vi "CloseBling.vi"(5 "Turn off LEDs on close":bool=TRUE, 8 "error in (no error)":errorcluster, 11 "ControlState in":T1 {"ChainMask" format="0x%02x"}) -> (0 "error out":errorcluster)   [LabVIEW 2020, in "ArduinoSerialBling.lvlib"]
uses:
  ArduinoSerialBling.lvlib
  ControlState.ctl
  ChainState.ctl
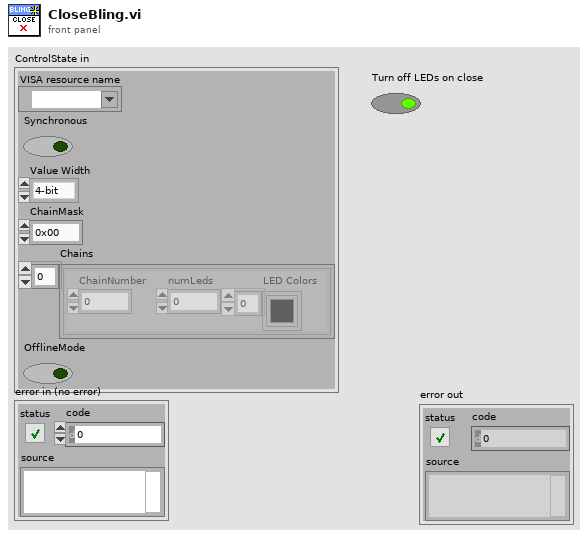
[diagram p1: front panel]
types:
  T1 = typedef "ArduinoSerialBling.lvlib/ControlState.ctl" = cluster{"VISA resource name":refnum<visa-resource-name>, "Synchronous":bool, "Value Width":enum16{"4-bit", "8-bit"}, "ChainMask":u8, "Chains":T2[], "OfflineMode":bool}
  T2 = typedef "ArduinoSerialBling.lvlib/ChainState.ctl" = cluster{"ChainNumber":u8, "numLeds":u8, "LED Colors":u32[]}
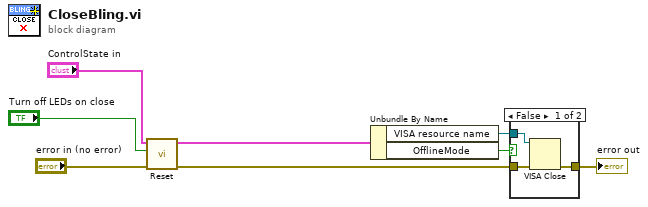
[diagram p0: block diagram]
diagram:
  n1 = call "Reset.vi"("error in (no error)"="error in (no error)", "Reset"="Turn off LEDs on close", "ControlState in"="ControlState in") -> ("error out"=w2:errorcluster, "ControlState out"=w3:T1)  [unwired: 7 in]
  n2 = Unbundle By Name(w3) -> ("VISA resource name"=w8:refnum<visa-resource-name>, "OfflineMode"=w6:bool)
  n3 = case shown="False" w6 {
    tunnel: w8 -> [w11 _]
    tunnel: w2 -> [w10 w12]
    tunnel: [w9 w12] -> w7
    frame False {
      n4 = VISA Close(VISA resource name=w11, error in (no error)=w10) -> (error out=w9:errorcluster)
    }
    frame True {
    }
  }
  "error out" <- w7
